vi "Get Channel Indices.vi"(10 "Task Structure":T1) -> (2 "Channel Indices":i32[](array[numeric]))   [LabVIEW 2020]
uses:
  Type Defs/Task Struct.ctl
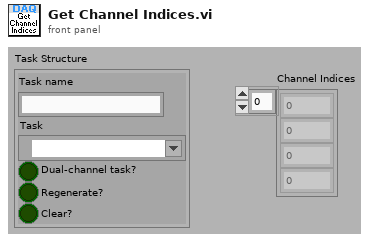
[diagram p1: front panel]
types:
  T1 = typedef "Task Struct.ctl" = cluster{"Task name":string, "Task":refnum<k21>, "Dual-channel task?":bool, "Regenerate?":bool, "Clear?":bool}
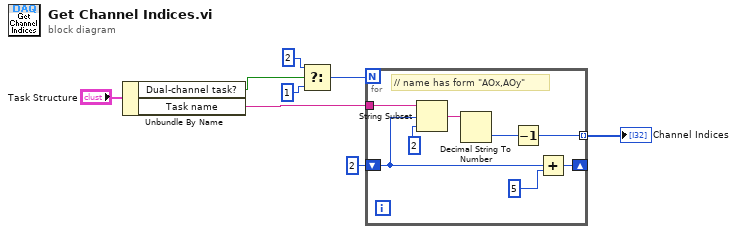
[diagram p0: block diagram]
diagram:
  n1 = Unbundle By Name("Task Structure") -> ("Dual-channel task?"=w4:bool, "Task name"=w5:string)
  n2 = Select(t=2, s=w4, f=1) -> (s? t:f=w1:i32)
  n3 = for {
    N: w1 -> [_]
    tunnel: w5 -> [w16]
    shift-right: [w14] -> _
    shift-left: 2 -> [w12]
    tunnel: [w9] -> w7 mode=indexing
    # "// name has form \"AOx,AOy\""
    n4 = String Subset(string=w16, offset (0)=w12, length (rest)=2 ("length (rest)")) -> (substring=w11:string)
    n5 = Decimal String To Number(string=w11) -> (number=w10:i32)  [unwired: 2 in, 1 out]
    n6 = Decrement(x=w10) -> (x-1=w9:i32)
    n7 = Add(x=w12, y=5) -> (x+y=w14:i32)
  }
  "Channel Indices" <- w7
